vi "(11) part 2 que.vi"() -> ()   [LabVIEW 2025]
panel:
  in  "length (len. of substring)":i32
  in  "offset (0)":i32
  in  "substring (\"\")":string
  in  "string":string
  out "result string":string
  # "it calculates the how much words to if we print 6 so in \ntop it selects 6 digits"
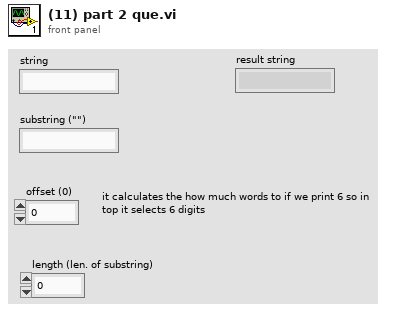
[diagram p1: front panel]
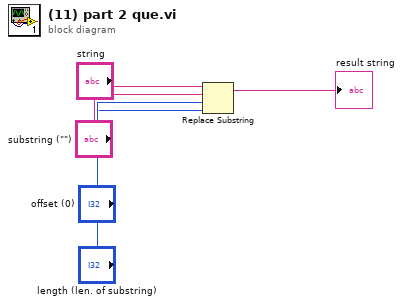
[diagram p0: block diagram]
diagram:
  n1 = Replace Substring(2:"length (len. of substring)", 3:"offset (0)", 4:"substring (\"\")", 5:"string") -> (1:→"result string":string)  [unwired: 1 out]
